vi "Duplicate.vi"(8 "error in":errorcluster, 10 "parameters":variant, 11 "Scope Instrument":refnum<class "Scope Instrument.lvclass">) -> (0 "error out":errorcluster, 3 "Scope Instrument out":refnum<class "Scope Instrument.lvclass">)   [LabVIEW 2025, in "Scope.lvlib" / "Scope Instrument.lvclass"]
doc: "Implements the specific behavior of a node when it is being duplicated\nCan be used to change the name of the new node for example adding Copy to it. \nCopyright 2017 National Instruments Corporation\n\nLicensed under the Apache License, Version 2.0 (the \"License\"); you may not use this file except in compliance with the License. You may obtain a copy of the License at http://www.apache.org/licenses/LICENSE-2.0\nUnless required by applicable law or agreed to in writing, software distributed under the License is distributed on an \"AS IS\" BASIS, WITHOUT WARRANTIES OR CONDITIONS OF ANY KIND, either express or implied. See the License for the specific language governing permissions and limitations under the License."
uses:
  Scope Instrument.lvclass
  Scope Instrument.lvclass/Scope Instrument.ctl
  Scope configuration/Scope configuration.lvclass
  C:/Users/Public/Documents/Sandia National Labs/TSS Plugin/Abstract Engine.lvlibp/Plugin/Abstract/Instrument configuration/Instrument configuration.lvclass
  Users/Public/Documents/Sandia National Labs/TSS Plugin/Abstract Engine.lvlibp/Plugin/Abstract/Instrument configuration/Read Instrument Setting.vi
  Users/Public/Documents/Sandia National Labs/TSS Plugin/Abstract Engine.lvlibp/Plugin/Abstract/Instrument configuration/Write Instrument Setting.vi
  Users/Public/Documents/Sandia National Labs/TSS Plugin/Abstract Engine.lvlibp/Plugin/Abstract/Abstract Instrument/Abstract Instrument.lvclass
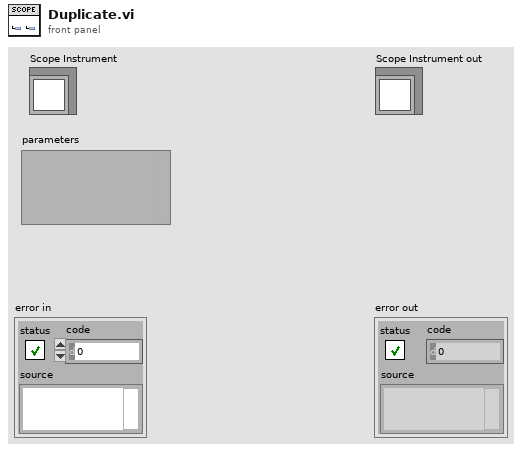
[diagram p1: front panel]
types:
  T1 = typedef "Abstract Engine.lvlibp/Instrument configuration.lvclass/Default Instrument.ctl" = cluster{"Type":string, "Address":string, "SW Alias":string, "Description":string, "Enabled":bool}
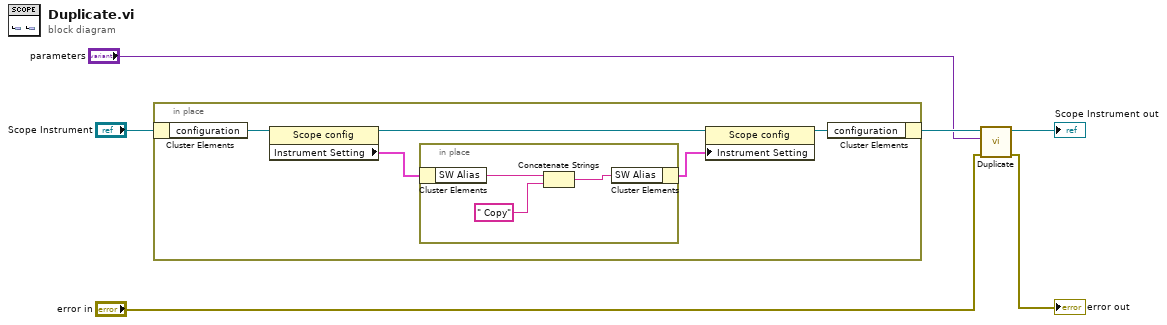
[diagram p0: block diagram]
diagram:
  n1 = in-place {
    n2 = in-place-cluster #1("Scope Instrument") -> ("configuration"=w11:refnum<class "Scope configuration.lvclass">)
    n3 = property class="Scope config"(reference=w11) -> (reference out=w9:refnum<class "Scope configuration.lvclass">, "Instrument Setting"=w8:T1)  [unwired: 1 in, 1 out]
    n4 = in-place {
      n5 = in-place-cluster #2(w8) -> ("SW Alias"=w14:string)
      n6 = Concatenate Strings(w14, " Copy") -> (w13:string)
      n7 = in-place-cluster #2("SW Alias"=w13) -> (w7:T1)
    }
    n8 = property class="Scope config"(reference=w9, "Instrument Setting"=w7) -> (reference out=w10:refnum<class "Scope configuration.lvclass">)  [unwired: 1 in, 1 out]
    n9 = in-place-cluster #1("configuration"=w10) -> (w4:refnum<class "Scope Instrument.lvclass">)
  }
  n10 = call-parent "Duplicate.vi"("error in"="error in", "parameters"="parameters", "CEF_Serialize node in"=w4) -> ("error out"=→"error out":errorcluster, "CEF_Serialize node out"=→"Scope Instrument out":refnum<class "Scope Instrument.lvclass">)  [unwired: 7 in]
